vi "Send subfolder levels.vi"(8 "error in (no error)":errorcluster, 11 "ImageStack in":refnum<class "ImageStack.lvclass">) -> (0 "error out":errorcluster, 3 "ImageStack out":refnum<class "ImageStack.lvclass">)   [LabVIEW 2012, in "ImageStack.lvclass"]
uses:
  ImageStack.lvclass
  <vilib>/Distrio/Murmex/Murmex/update_cluster.ctl
  <vilib>/Distrio/Murmex/Murmex/Murmex.lvclass
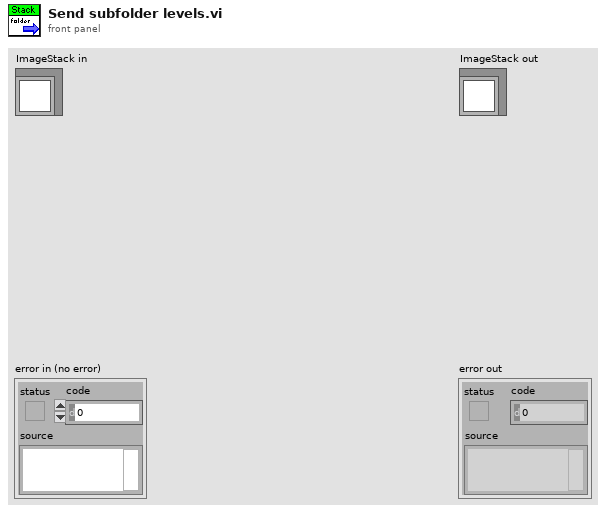
[diagram p1: front panel]
types:
  T1 = typedef "Murmex.lvlib/Murmex.lvclass/update_cluster.ctl" = cluster{"target ID":string, "key chains":string[], "values":variant[]}
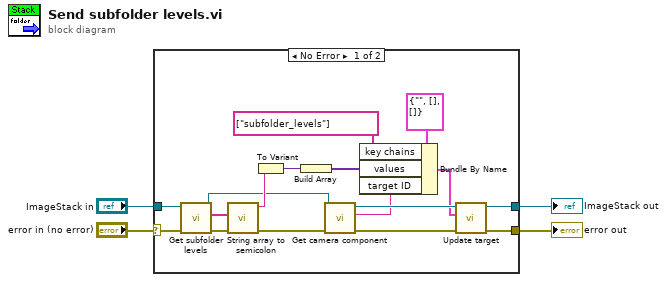
[diagram p0: block diagram]
diagram:
  n1 = case shown="No Error" "error in (no error)" {
    selector: "error in (no error)" -> [w14 w23]
    tunnel: [w21 w23] -> w3
    tunnel: [w17 w22] -> w1
    tunnel: "ImageStack in" -> [w15 w22]
    frame No Error {
      n2 = call-dynamic "Get subfolder levels.vi"("error in (no error)"=w14, "ImageStack in"=w15) -> ("error out"=w13:errorcluster, "Subfolder levels"=w9:string[], "ImageStack out"=w8:refnum<class "ImageStack.lvclass">)  [unwired: 7 in]
      n3 = call "String array to semicolon.vi"("error in"=w13, "String array"=w9) -> ("error out"=w12:errorcluster, "Semicolon string"=w11:string)  [unwired: 8 in]
      n4 = To Variant(anything=w11) -> (Variant=w10:variant)
      n5 = Build Array(w10) -> (w6:variant[])
      n6 = call-dynamic "Get camera component.vi"("error in (no error)"=w12, "ImageStack in"=w8) -> ("error out"=w19:errorcluster, "Camera component name"=w5:string, "ImageStack out"=w18:refnum<class "ImageStack.lvclass">)  [unwired: 7 in]
      n7 = Bundle By Name(cluster=T1 {"target ID"="", "key chains"=[], "values"=[]} ("update cluster"), "key chains"=string[] ["subfolder_levels"], "values"=w6, "target ID"=w5) -> (w7:T1)
      n8 = call <vilib>:"Update target.vi"("error in (no error)"=w19, "update cluster"=w7, "MurmexBase in"=w18) -> ("error out"=w21:errorcluster, "MurmexBase out"=w17:refnum<class "ImageStack.lvclass">)  [unwired: 7 in]
    }
    frame Error {
    }
  }
  "error out" <- w3
  "ImageStack out" <- w1
